vi "Lakeshore 331 Configure Parameters GUI.vi"(11 "Temp Control Parms":T1={"Mode"=2, "Setpoint"=0.0, "Manual Power (%)"=0.0, "Control Parameters"={"P"=0.0, "I"=0.0, "D"=0}, "Heater Range"=0, "Default Range"=0} {"Default Range" items=["Off", "Low (0.5W)", "Med (5W)", "High (50W)"]; "Heater Range" items=["Off", "Low (0.5W)", "Med (5W)", "High (50W)"]; "Manual Power (%)" format="%.3f"; "Mode" items=["Manual PID"=1, "Zone"=2, "Open Loop"=3, "AutoTune PID"=4, "AutoTune PI"=5, "AutoTune P"=6]}) -> (2 "Cancelled":bool, 3 "Temp Control Parms out":T1={"Mode"=2, "Setpoint"=0.0, "Manual Power (%)"=0.0, "Control Parameters"={"P"=0.0, "I"=0.0, "D"=0}, "Heater Range"=0, "Default Range"=0} {"Default Range" items=["Off", "Low (0.5W)", "Med (5W)", "High (50W)"]; "Heater Range" items=["Off", "Low (0.5W)", "Med (5W)", "High (50W)"]; "Manual Power (%)" format="%.3f"; "Mode" items=["Manual PID"=1, "Zone"=2, "Open Loop"=3, "AutoTune PID"=4, "AutoTune PI"=5, "AutoTune P"=6]})   [LabVIEW 2022 SP3, in "Lakeshore 331.lvclass"]
uses:
  Lakeshore 331.lvclass
  Temp Control Parameters.ctl
  Lakeshore 331.lvclass/Lakeshore 331.ctl
  Temp Control.lvclass
panel:
  in  "Cancel Button":bool
  in  "OK Button":bool
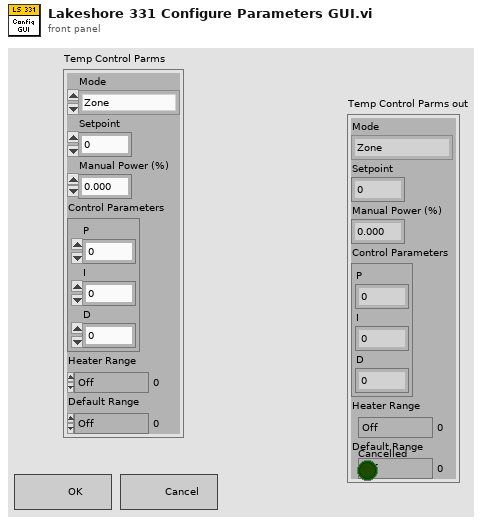
[diagram p1: front panel]
types:
  T1 = typedef "Temp Control.lvclass/Temp Control Parameters.ctl" = cluster{"Mode":u16, "Setpoint":dbl, "Manual Power (%)":dbl, "Control Parameters":cluster{"P":dbl, "I":dbl, "D":u16}, "Heater Range":u16, "Default Range":u16}
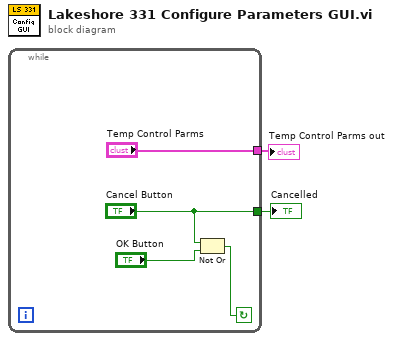
[diagram p0: block diagram]
diagram:
  n1 = while {
    tunnel: ["Temp Control Parms"] -> w2
    tunnel: ["Cancel Button"] -> w1
    stop <- w4 continue-if-true
    n2 = Not Or(1:"OK Button", 2:"Cancel Button") -> (0:w4:bool)
  }
  "Temp Control Parms out" <- w2
  "Cancelled" <- w1
